vi "Script gRPC.vi"(8 "error in":errorcluster, 10 "Generated Library Name":string, 11 "proto File Path":path) -> (0 "error out":errorcluster)   [LabVIEW 2021, in "Script gRPC.lvlib"]
uses:
  Script gRPC.lvlib
  <vilib>/CIF Foundation/CIF Core/CIFUtilities/CIFConfigurationFile/CIF Configuration File.lvlib
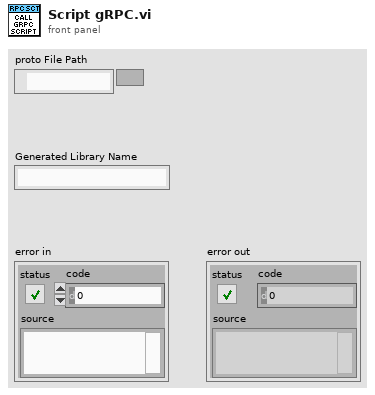
[diagram p1: front panel]
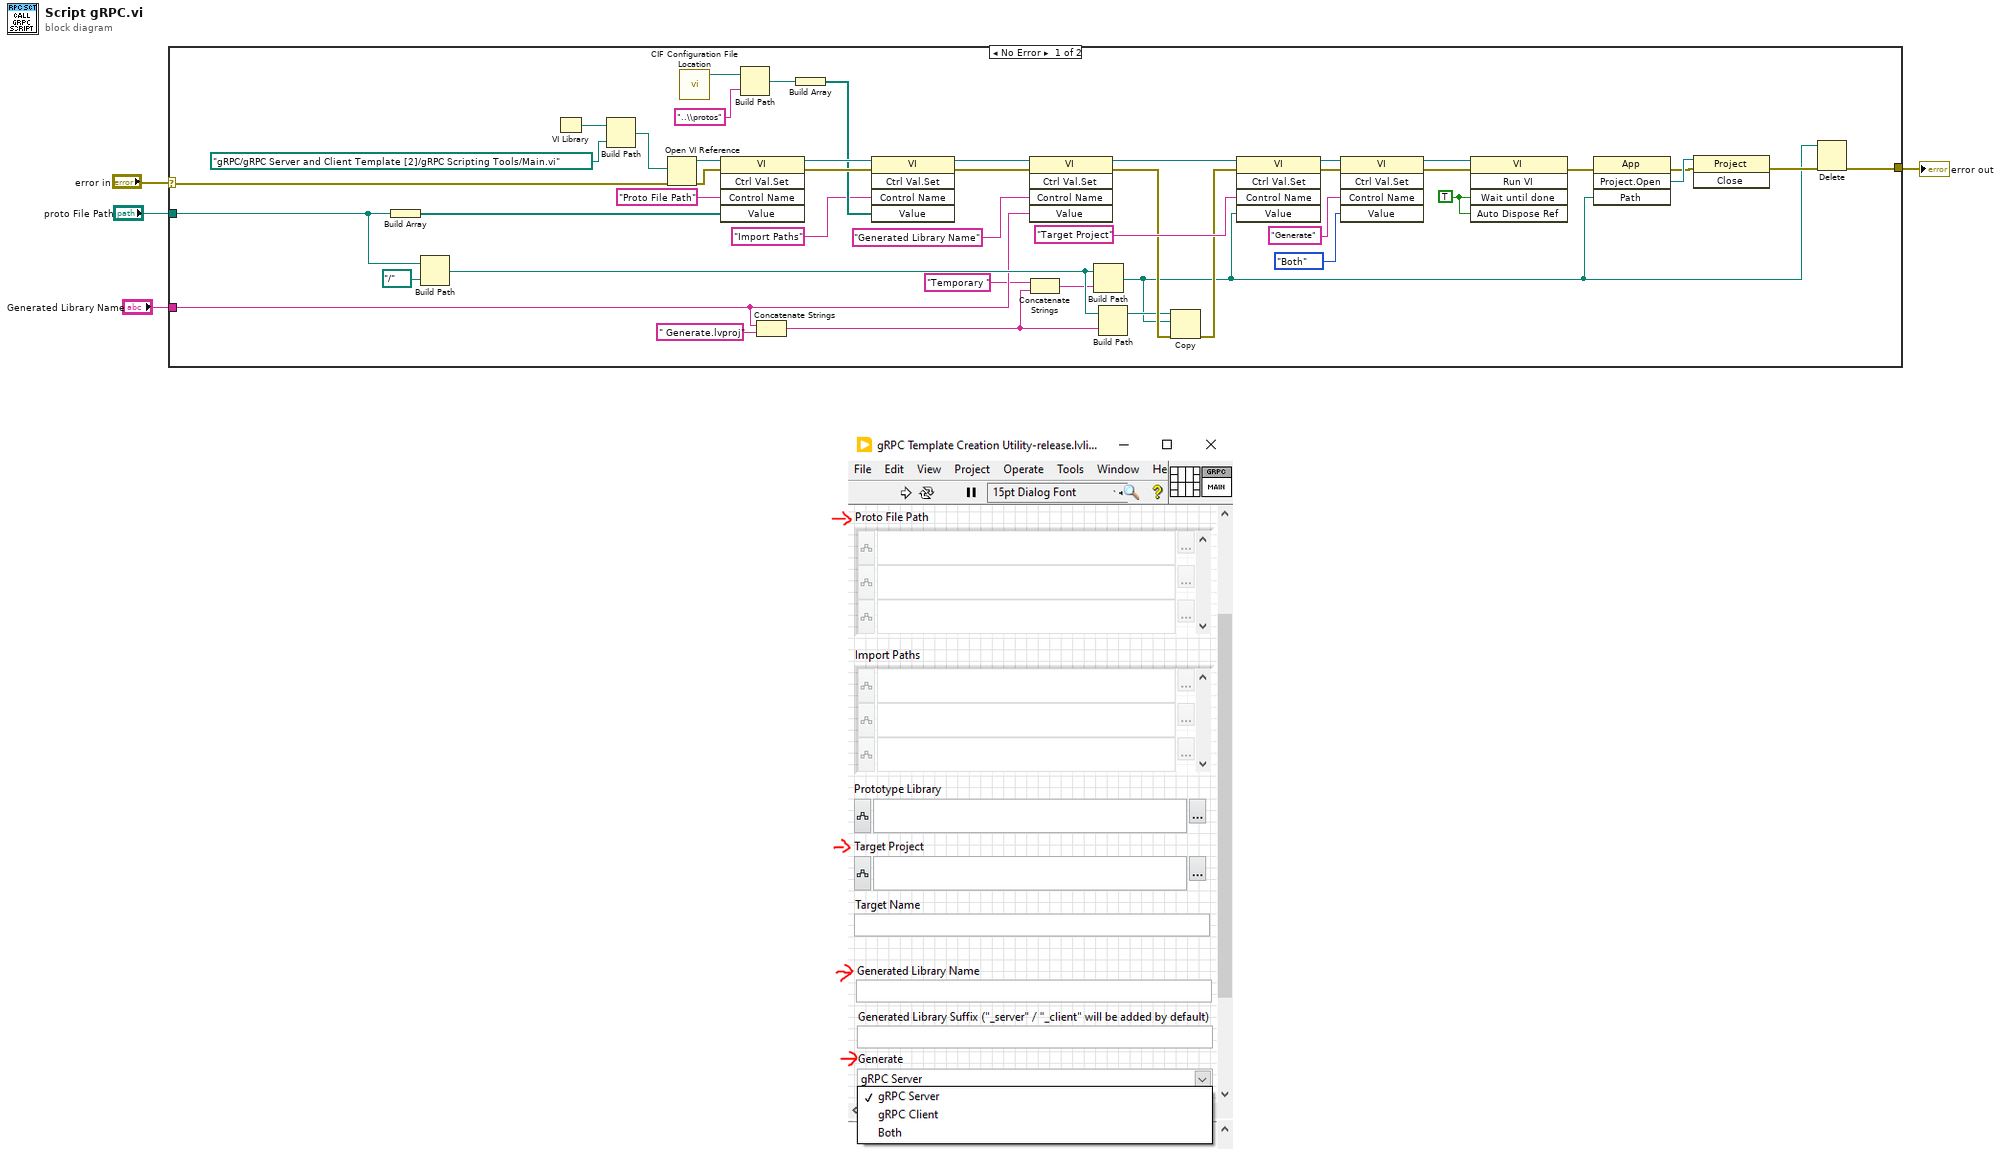
[diagram p0: block diagram]
diagram:
  n1 = case shown="No Error" "error in" {
    selector: "error in" -> [w20 w49]
    tunnel: [w24 w49] -> w4
    tunnel: "proto File Path" -> [w27 _]
    tunnel: "Generated Library Name" -> [w10 _]
    frame No Error {
      w28 = TRUE ("Wait Until Done")
      n2 = Build Array(w27) -> (w33:path[])
      n3 = Build Path(base path=w27, name or relative path=path "../..") -> (appended path=w25:path)
      n4 = VI Library() -> (path=w48:path)
      n5 = Build Path(base path=w48, name or relative path=path "gRPC/gRPC Server and Client Template [2]/gRPC Scripting Tools/Main.vi") -> (appended path=w46:path)
      n6 = Open VI Reference(vi path=w46, error in (no error)=w20) -> (vi reference=w35:refnum<vi>, error out=w34:errorcluster)  [unwired: 4 in]
      n7 = call <vilib>:"CIF Configuration File Location.vi"() -> ("configuration file path"=w15:path)  [unwired: 11 in]
      n8 = invoke class="VI" method="Ctrl Val.Set"(reference=w35, error in=w34, "Control Name"="Proto File Path", "Value"=w33) -> (reference out=w19:refnum<vi>, error out=w18:errorcluster)  [unwired: 1 in, 3 out]
      n9 = Build Path(base path=w15, name or relative path="..\\protos" ("Control Name")) -> (appended path=w13:path)
      n10 = Concatenate Strings(w10, " Generate.lvproj" ("string")) -> (w8:string)
      n11 = Build Array(w13) -> (w12:path[])
      n12 = invoke class="VI" method="Ctrl Val.Set"(reference=w19, error in=w18, "Control Name"="Import Paths", "Value"=w12) -> (reference out=w17:refnum<vi>, error out=w16:errorcluster)  [unwired: 1 in, 3 out]
      n13 = invoke class="VI" method="Ctrl Val.Set"(reference=w17, error in=w16, "Control Name"="Generated Library Name", "Value"=w10) -> (reference out=w43:refnum<vi>, error out=w23:errorcluster)  [unwired: 1 in, 3 out]
      n14 = Concatenate Strings("Temporary " ("string"), w8) -> (w5:string)
      n15 = Build Path(base path=w25, name or relative path=w5) -> (appended path=w6:path)
      n16 = Build Path(base path=w25, name or relative path=w8) -> (appended path=w7:path)
      n17 = Copy(8:w23, 10:w6, 11:w7) -> (0:w22:errorcluster)  [unwired: 2 in, 2 out]
      n18 = invoke class="VI" method="Ctrl Val.Set"(reference=w43, error in=w22, "Control Name"="Target Project", "Value"=w6) -> (reference out=w41:refnum<vi>, error out=w40:errorcluster)  [unwired: 1 in, 3 out]
      n19 = invoke class="VI" method="Ctrl Val.Set"(reference=w41, error in=w40, "Control Name"="Generate", "Value"=enum16{"gRPC Server", "gRPC Client", "Both"}."Both" ("Generate")) -> (reference out=w37:refnum<vi>, error out=w36:errorcluster)  [unwired: 1 in, 3 out]
      n20 = invoke class="VI" method="Run VI"(reference=w37, error in=w36, "Wait until done"=w28, "Auto Dispose Ref"=w28) -> (error out=w29:errorcluster)  [unwired: 1 in, 4 out]
      n21 = invoke class="App" method="Project.Open"(error in=w29, "Path"=w6) -> (error out=w30:errorcluster, "Project:Open"=w31:refnum<vi>)  [unwired: 2 in, 2 out]
      n22 = invoke class="Project" method="Close"(reference=w31, error in=w30) -> (error out=w21:errorcluster)  [unwired: 1 in, 2 out]
      n23 = Delete(path (use dialog)=w6, error in=w21) -> (error out=w24:errorcluster)  [unwired: 3 in, 2 out]
    }
    frame Error {
    }
  }
  "error out" <- w4
